vi "Robot Global Data.vi"() -> ()   [LabVIEW 2011]
doc: "This global VI can contain as many global variables as you need. Place a control on the panel, give it a good name. To read or write to it from a VI, drag the icon to the diagram of that VI. You can also drag from the project. Click on the node to change which global you access. You shouldn't have multiple locations writing to a global or it will cause a race-condition."
uses:
  <vilib>/Rock Robotics/WPI/Camera/WPI_CameraImageSize.ctl
panel:
  out "Wheel Encoder Reset":bool
  out "Robot Angle":dbl(knob) scale=0.0..10.0
  out "Turntable Angle":dbl(knob) scale=0.0..360.0
  out "Aim Angle Y":dbl(knob) scale=0.0..360.0
  out "Aim Angle X":dbl(knob) scale=0.0..360.0
  out "Camera Distance":dbl
  out "Camera Y":dbl
  out "Camera X":dbl
  out "RPM Indicator":dbl
  out "RPM":dbl(knob) scale=0.0..4000.0
  out "Target Info":T1(array[cluster])
  out "Shoot angle":dbl
  out "Turntable Rate":dbl
  out "Turntable Distance":dbl
  out "Right Wheels Rate":dbl(knob) scale=0.0..2200.0
  out "Left Wheels Rate":dbl(knob) scale=0.0..2200.0
  out "Right Wheels Distance":dbl
  out "Left Wheels Distance":dbl
  out "units":string="inches"
  out "Sonar Distance":dbl(slide)=60.0 scale=0.0..120.0 scale format="%#.3g"
  out "Acceleration Z":dbl
  out "Acceleration Y":dbl
  out "Acceleration X":dbl
  out "Gyro Angle":dbl(knob) scale=0.0..360.0
  in  "LED toggle rate (ms)":u32=20
  in  "image size":T2=enum."320x240"
  in  "Enable Vision":bool
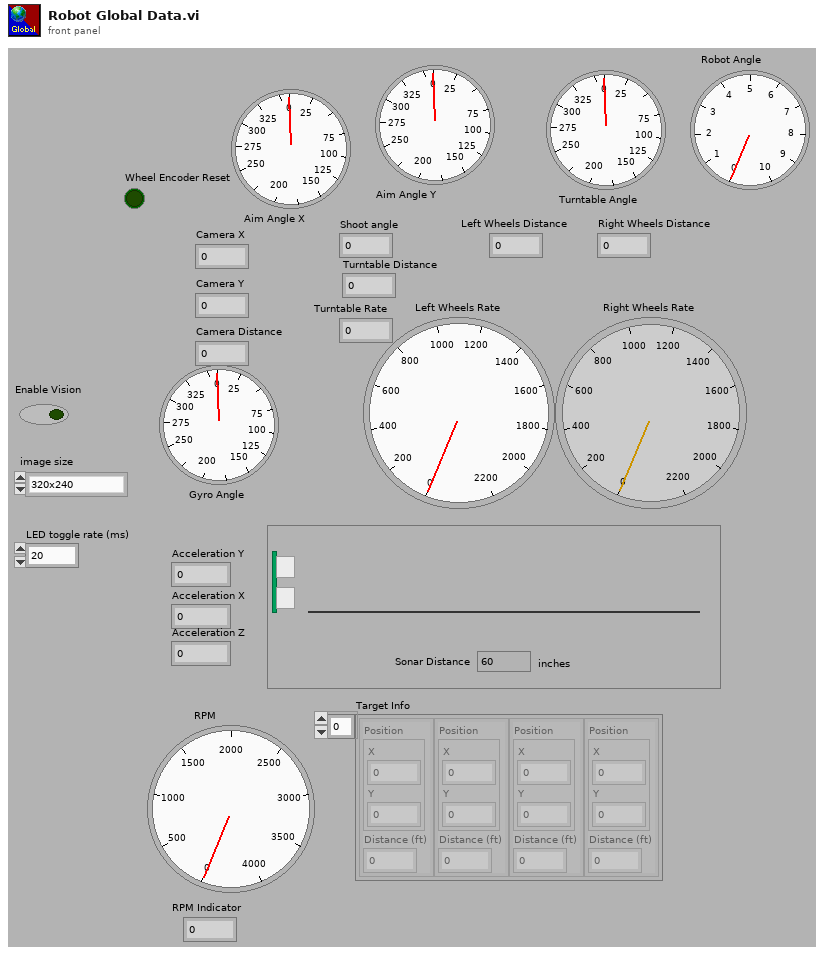
[diagram p1: front panel]
types:
  T1 = cluster{"Position":cluster{"X":dbl, "Y":dbl}, "Distance (ft)":dbl}[]
  T2 = typedef "WPI_CameraImageSize.ctl" = enum16{"640x480", "320x240", "160x120"}
diagram:
